vi "FindAnnularh.vi"(6 "Save Options":T1={"Save h Files?"=FALSE, "Save image data?"=FALSE, "Path"=path "E:/Test"}, 7 "Full h(r,t)":bool, 9 "Ring Number":i32, 10 "Variables in":T2={"Number of rings"=1, "sound spd (cm/s)"=150000, "z span (cm)"=4.0, "z steps"=20, "y span (cm)"=50.0, "y steps"=0, "time step (s)"=1e-08, "z"=0.0, "y"=0.0, "ref delay"=0.0, "freq (MHz)"=4.71, "cycles"=300} {"freq (MHz)" format="%.2f"; "z span (cm)" format="%.2f"; "y" format="%.2f"; "ref delay" format="%.2f"; "y span (cm)" format="%.2f"; "z" format="%.2f"; "time step (s)" format="%.2e"}, 11 "Annular rings":cluster{"Radius":dbl, "a":dbl}[](array[cluster]) {"a" format="%.2f"; "Radius" format="%.2f"}) -> (0 "Y axis":dbl[](array[numeric]) format="%.2f", 3 "h(r,t)":dbl[][](array[numeric]) format="%.2f", 5 "delay pts":i32[](array[numeric]))   [LabVIEW 2022 SP3]
uses:
  <vilib>/Math Plots/3D Math Plots/3D Surface/3D Surface XCtrl/3D Surface.xctl
  <vilib>/Math Plots/3D Math Plots/3D Surface/3D Surface Datatype/Public/Plot Helper (Matrix).vi
  <vilib>/Math Plots/3D Math Plots/3D Surface/3D Surface Datatype/3D Surface Datatype.lvclass
panel:
  out "3D Surface":refnum<class "3D Plot Datatype.lvclass">[](xcontrol)
  in  "Display 3-D?":bool
  in  "Index (row)":i32
  out "view h(r,t)":dbl[](graph)
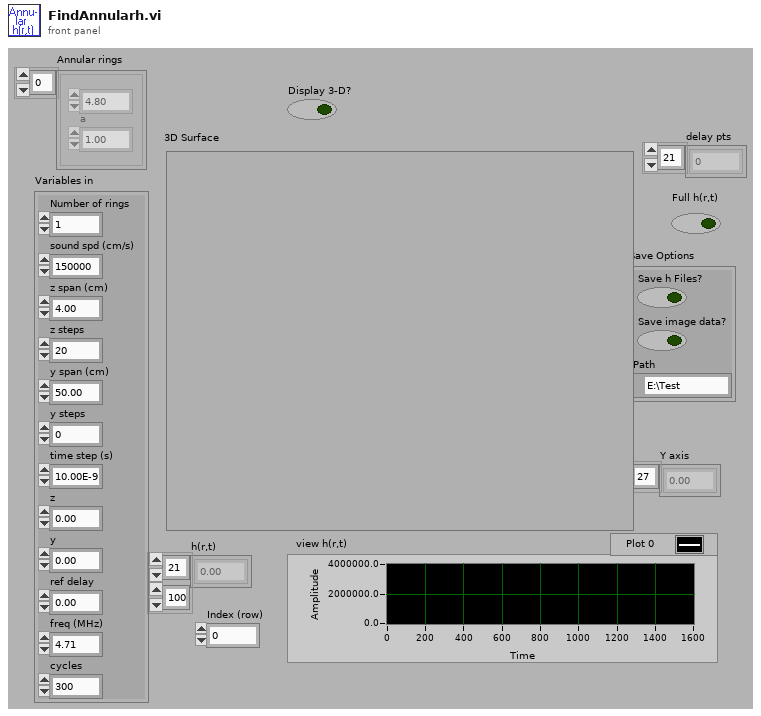
[diagram p1: front panel]
types:
  T1 = cluster{"Save h Files?":bool, "Save image data?":bool, "Path":path}
  T2 = cluster{"Number of rings":i32, "sound spd (cm/s)":i32, "z span (cm)":dbl, "z steps":i32, "y span (cm)":dbl, "y steps":i32, "time step (s)":sgl, "z":dbl, "y":dbl, "ref delay":dbl, "freq (MHz)":dbl, "cycles":i32}
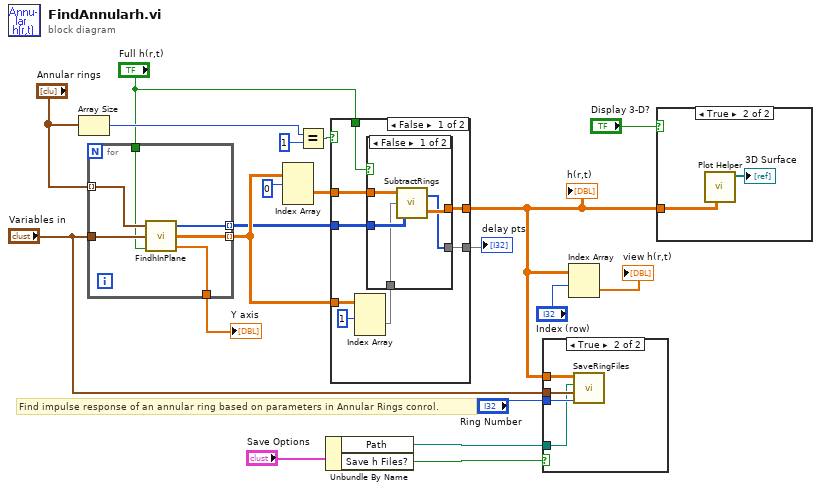
[diagram p0: block diagram]
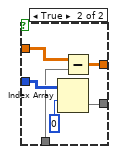
[diagram p4: hidden frame]
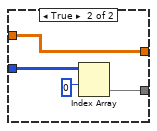
[diagram p5: hidden frame]
diagram:
  # "Find impulse response of an annular ring based on parameters in Annular Rings conrol."
  n1 = Array Size(array="Annular rings") -> (size(s)=w16:i32)
  n2 = for {
    tunnel: [w26] -> w5 mode=indexing
    tunnel: "Variables in" -> [w24]
    tunnel: "Annular rings" -> [w25] mode=indexing
    tunnel: [w23] -> w11
    tunnel: [w22] -> w1 mode=indexing
    tunnel: "Full h(r,t)" -> [w21]
    n3 = call "FindhInPlane.vi"("Full h(r,t)"=w21, "Variables in"=w24, "Trans Geometry"=w25) -> ("Y axis"=w23:dbl[], "h(r,t)"=w26:dbl[][], "delay pts"=w22:i32[])
  }
  "Y axis" <- w11
  n4 = Index Array(array=w5, index (dim 0)=0) -> (element=w19:dbl[][])  [unwired: 2 in]
  n5 = Equal?(x=w16, y=1) -> (x = y?=w17:bool)
  n6 = Unbundle By Name("Save Options") -> ("Path"=w7:path, "Save h Files?"=w8:bool)
  n7 = case shown="False" w17 {
    tunnel: w19 -> [w27 w46]
    tunnel: [w34 w46] -> w3
    tunnel: w5 -> [w32 _]
    tunnel: w1 -> [w28 w47]
    tunnel: "Full h(r,t)" -> [w31 _]
    tunnel: [w30 w48] -> w2
    frame False {
      n8 = Index Array(array=w32, index (dim 0)=1) -> (element=w29:dbl[][])  [unwired: 2 in]
      n9 = case shown="False" w31 {
        tunnel: w27 -> [w38 w43]
        tunnel: [w36 w41] -> w34
        tunnel: w29 -> [w37 w42]
        tunnel: w28 -> [w39 w44]
        tunnel: [w35 w40] -> w30
        frame False {
          n10 = call "SubtractRings.vi"("delay pts"=w39, "h(r,t) ring inner"=w37, "h(r,t) ring outer"=w38) -> ("h(r,t) annulus"=w36:dbl[][], "delay pts out"=w35:i32[])
        }
        frame True {
          n11 = Index Array(array=w44, index (row)=0) -> (element=w40:i32[])  [unwired: 1 in]
          n12 = Subtract(x=w43, y=w42) -> (x-y=w41:dbl[][])
        }
      }
    }
    frame True {
      n13 = Index Array(array=w47, index (row)=0) -> (element=w48:i32[])  [unwired: 1 in]
    }
  }
  "h(r,t)" <- w3
  "delay pts" <- w2
  n14 = case shown="True" w8 {
    tunnel: "Ring Number" -> [_ w53]
    tunnel: w3 -> [_ w52]
    tunnel: "Variables in" -> [_ w51]
    tunnel: w7 -> [_ w50]
    frame False {
    }
    frame True {
      n15 = call "SaveRingFiles.vi"("h(r,t)"=w52, "Path"=w50, "Variables in"=w51, "Ring Number"=w53) -> ()  [unwired: 1 in, 4 out]
    }
  }
  n16 = Index Array(array=w3, index (row)="Index (row)") -> (element=→"view h(r,t)":dbl[])  [unwired: 1 in]
  n17 = case shown="True" "Display 3-D?" {
    tunnel: w3 -> [_ w54]
    frame False {
    }
    frame True {
      n18 = call-poly <vilib>:"Plot Helper.vi"("z matrix"=w54) -> ("3D Plot lvclass Array out"=→"3D Surface":refnum<class "3D Plot Datatype.lvclass">[])  [unwired: 5 in, 5 out]
    }
  }
